vi "midi_OpenInstruments.vi"(8 "error in (no error)":errorcluster, 9 "mute":bool[](array[boolean]), 10 "preview":bool[](array[boolean]), 11 "instruments":path[](array[path])=[path "", path "", path "", path "", path "", path "", path "", path "", path "", path "", path "", path "", path "", path "", path "", path ""]) -> (0 "error out":errorcluster, 3 "vi references":refnum<vi>[](array[refnum]))   [LabVIEW 2013]
doc: "Open the \"instrument\" subVIs that comprise \"The Band.\""
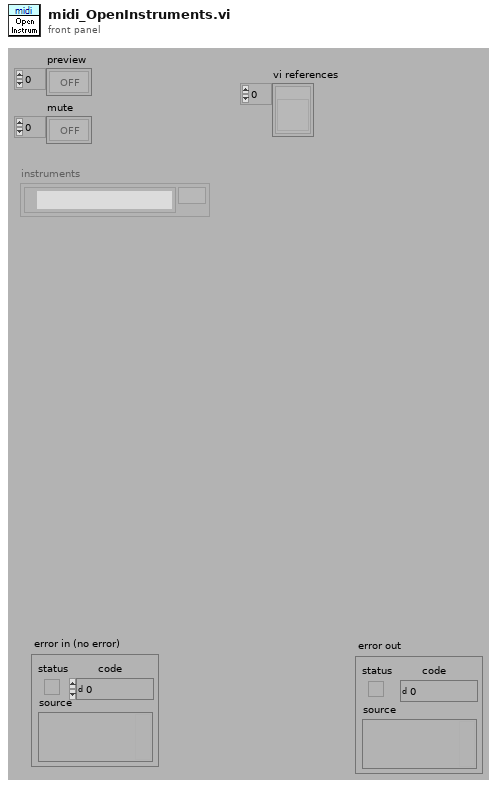
[diagram p1: front panel]
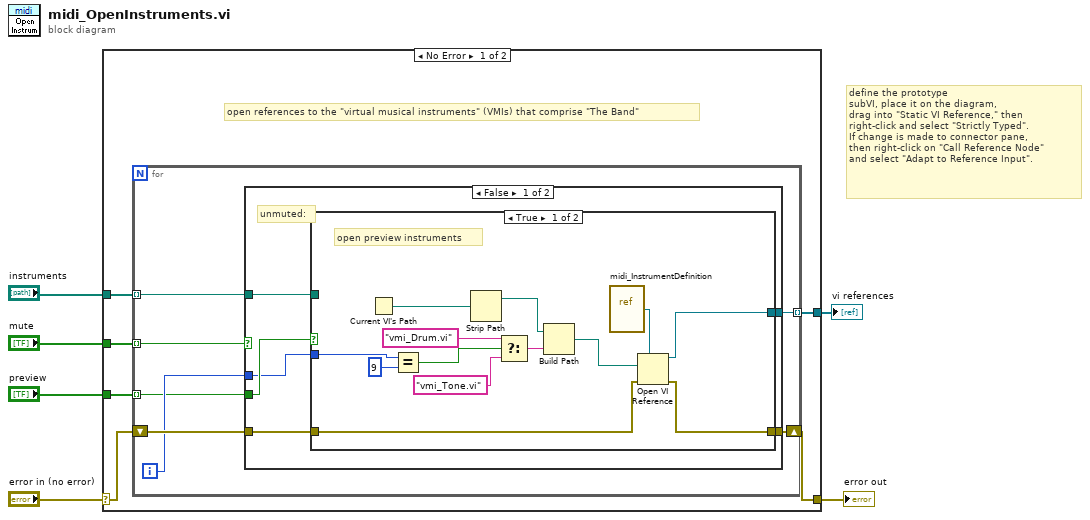
[diagram p0: block diagram]
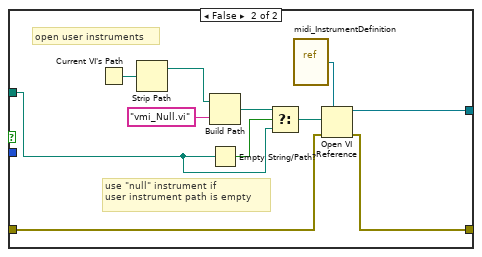
[diagram p2: hidden frame]
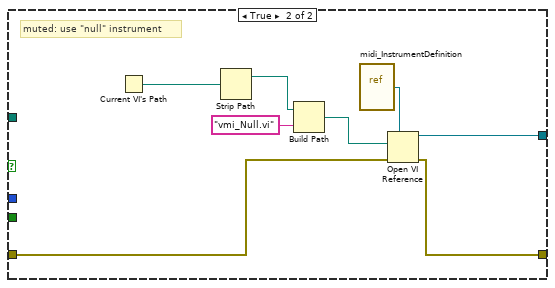
[diagram p3: hidden frame]
diagram:
  # "define the prototype\nsubVI, place it on the diagram,\ndrag into \"Static VI Reference,\" then\nright-click and select \"Strictly Typed\".\nIf change is made to connector pane,\nthen right-click on \"Call Reference Node\"\nand select \"Adapt to Reference Input\"."
  n1 = case shown="No Error" "error in (no error)" {
    selector: "error in (no error)" -> [w12 w58]
    tunnel: [w11 w58] -> w5
    tunnel: [w10 _] -> w4
    tunnel: "mute" -> [w9 _]
    tunnel: "instruments" -> [w8 _]
    tunnel: "preview" -> [w7 _]
    frame No Error {
      # "open references to the \"virtual musical instruments\" (VMIs) that comprise \"The Band\""
      n2 = for {
        tunnel: [w17] -> w10 mode=indexing
        shift-right: [w18] -> w11
        shift-left: w12 -> [w19]
        tunnel: w9 -> [w14] mode=indexing
        tunnel: w8 -> [w15] mode=indexing
        tunnel: w7 -> [w13] mode=indexing
        i -> [w16]
        n3 = case shown="False" w14 {
          tunnel: w19 -> [w25 w55]
          tunnel: [w24 w54] -> w18
          tunnel: [w23 w53] -> w17
          tunnel: w16 -> [w20 _]
          tunnel: w15 -> [w22 _]
          tunnel: w13 -> [w21 _]
          frame False {
            # "unmuted:"
            n4 = case shown="True" w21 {
              tunnel: w25 -> [w29 w49]
              tunnel: [w28 w48] -> w24
              tunnel: [w27 w47] -> w23
              tunnel: w22 -> [_ w39]
              tunnel: w20 -> [w26 _]
              frame True {
                # "open preview instruments"
                n5 = Current VI's Path() -> (path=w36:path)
                n6 = Equal?(x=w26, y=9) -> (x = y?=w31:bool)
                n7 = Strip Path(path=w36) -> (stripped path=w35:path)  [unwired: 1 out]
                n8 = Select(t="vmi_Drum.vi" ("string"), s=w31, f="vmi_Tone.vi" ("string")) -> (s? t:f=w30:string)
                n9 = Build Path(base path=w35, name or relative path=w30) -> (appended path=w37:path)
                n10 = vi-ref "midi_InstrumentDefinition.vi"() -> (w38:refnum<vi>)
                n11 = Open VI Reference(type specifier VI Refnum (for type only)=w38, vi path=w37, error in (no error)=w29) -> (vi reference=w27:refnum<vi>, error out=w28:errorcluster)  [unwired: 3 in]
              }
              frame False {
                # "use \"null\" instrument if\nuser instrument path is empty"
                # "open user instruments"
                n12 = Current VI's Path() -> (path=w45:path)
                n13 = Strip Path(path=w45) -> (stripped path=w44:path)  [unwired: 1 out]
                n14 = Build Path(base path=w44, name or relative path="vmi_Null.vi" ("string")) -> (appended path=w42:path)
                n15 = Empty String/Path?(string/path=w39) -> (empty?=w41:bool)
                n16 = Select(t=w42, s=w41, f=w39) -> (s? t:f=w40:path)
                n17 = vi-ref "midi_InstrumentDefinition.vi"() -> (w46:refnum<vi>)
                n18 = Open VI Reference(type specifier VI Refnum (for type only)=w46, vi path=w40, error in (no error)=w49) -> (vi reference=w47:refnum<vi>, error out=w48:errorcluster)  [unwired: 3 in]
              }
            }
          }
          frame True {
            # "muted: use \"null\" instrument"
            n19 = Current VI's Path() -> (path=w52:path)
            n20 = Strip Path(path=w52) -> (stripped path=w51:path)  [unwired: 1 out]
            n21 = Build Path(base path=w51, name or relative path="vmi_Null.vi" ("string")) -> (appended path=w56:path)
            n22 = vi-ref "midi_InstrumentDefinition.vi"() -> (w57:refnum<vi>)
            n23 = Open VI Reference(type specifier VI Refnum (for type only)=w57, vi path=w56, error in (no error)=w55) -> (vi reference=w53:refnum<vi>, error out=w54:errorcluster)  [unwired: 3 in]
          }
        }
      }
    }
    frame Error {
    }
  }
  "error out" <- w5
  "vi references" <- w4
